vi "LJUD_OpenLabJack.vi"(6 "FirstFound":bool=TRUE, 7 "Address":string="192.168.1.209", 8 "error in":errorcluster, 9 "ConnectionType":i32=2, 10 "DeviceType":i32=9) -> (0 "error out":errorcluster, 3 "Handle":i32)   [LabVIEW 2020]
doc: "Call an Open function to get a handle to a device. That handle\nis then passed to other functions to write & read values.\n\nDocumented in Section 4.2 of the device's datasheet, with further\ninformation in Section 4.3.\n\nDeviceType: LJ_dtU3=3, LJ_dtU6=6, LJ_dtUE9=9\n\nConnectionType: LJ_ctUSB=1, LJ_ctETHERNET=2\n\nAddress: For USB, pass the local ID or serial number of the desired\nLabJack. For Ethernet pass the IP address of the desired LabJack. If\nFirstFound is true, Address is ignored.\n\nFirstFound: If true, then the Address and ConnectionType parameters\nare ignored and the driver opens the first LabJack found with the\nspecified DeviceType. Generally only recommended when a single\nLabJack is connected. Currently only supported with USB. If a USB\ndevice is not found, it will try Ethernet but with the given Address."
uses:
  labjackud.dll
panel:
  # "Call an Open function to get a handle to a device.  That handle\nis then passed to other functions to write & read values.\n\nDocumented in Section 4.2 of the device's datasheet, with further\ninformation in Section 4.3.\n\nDeviceType:  LJ_dtU3=3, LJ_dtU6=6, LJ_dtUE9=9\n\nConnectionType:  LJ_ctUSB=1, LJ_ctETHERNET=2\n\nAddress:  For USB, pass the local ID or serial number of the desired\nLabJack. For Ethernet pass the IP address of the desired LabJack. If\nFirstFound is true, Address is ignored.\n\nFirstFound:  If true, then the Address and ConnectionType parameters\nare ignored and the driver opens the first LabJack found with the\nspecified DeviceType. Generally only recommended when a single\nLabJack is connected. Currently only supported with USB. If a USB\ndevice is not found, it will try Ethernet but with the given Address."
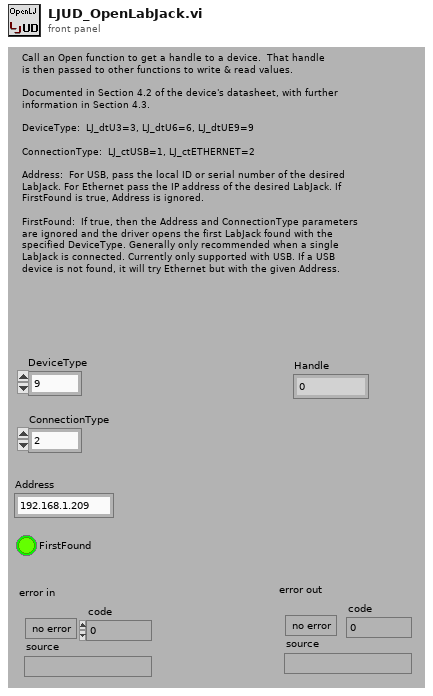
[diagram p1: front panel]
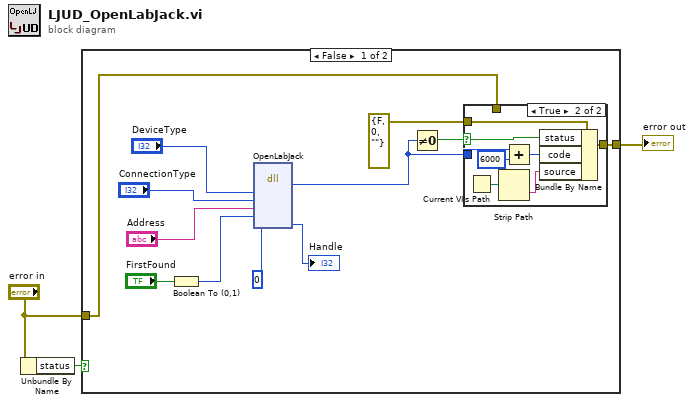
[diagram p0: block diagram]
diagram:
  n1 = Unbundle By Name("error in") -> ("status"=w2:bool)
  n2 = case shown="False" w2 {
    tunnel: [w5 w25] -> w3
    tunnel: "error in" -> [w4 w25]
    frame False {
      n3 = Boolean To (0,1)(Boolean="FirstFound") -> (0, 1=w11:i16)
      n4 = dll-call lib="labjackud.dll" fn="OpenLabJack"("DeviceType"="DeviceType", "ConnectionType"="ConnectionType", "Address"="Address", "FirstFound"=w11, "Handle"=0) -> (w6:i32, "Handle"=→"Handle":i32)  [unwired: 7 in, 2 out]
      n5 = Not Equal To 0?(x=w6) -> (x != 0?=w7:bool)
      n6 = case shown="True" w7 {
        selector: w7 -> [_ w23]
        tunnel: [w16 w24] -> w5
        tunnel: errorcluster {"status"=FALSE, "code"=0, "source"=""} ("error IO") -> [_ w22]
        tunnel: w6 -> [_ w18]
        tunnel: w4 -> [w16 _]
        frame False {
        }
        frame True {
          n7 = Current VI's Path() -> (path=w20:path)
          n8 = Strip Path(path=w20) -> (name=w21:string)  [unwired: 1 out]
          n9 = Add(x=w18, y=6000) -> (x+y=w19:i32)
          n10 = Bundle By Name(cluster=w22, "status"=w23, "code"=w19, "source"=w21) -> (w24:errorcluster)
        }
      }
    }
    frame True {
    }
  }
  "error out" <- w3
